vi "LookupFilepath.vi"(0 "Filepath Map":cluster{"Key":string, "Filepath":path}[](array[cluster]), 5 "FileID":string, 11 "error in":errorcluster) -> (15 "error out":errorcluster)   [LabVIEW 2014, in "LinksApplication.lvclass"]
uses:
  LinksApplication.lvclass
panel:
  # "Inputs"
  # "Debug"
  # "Outputs"
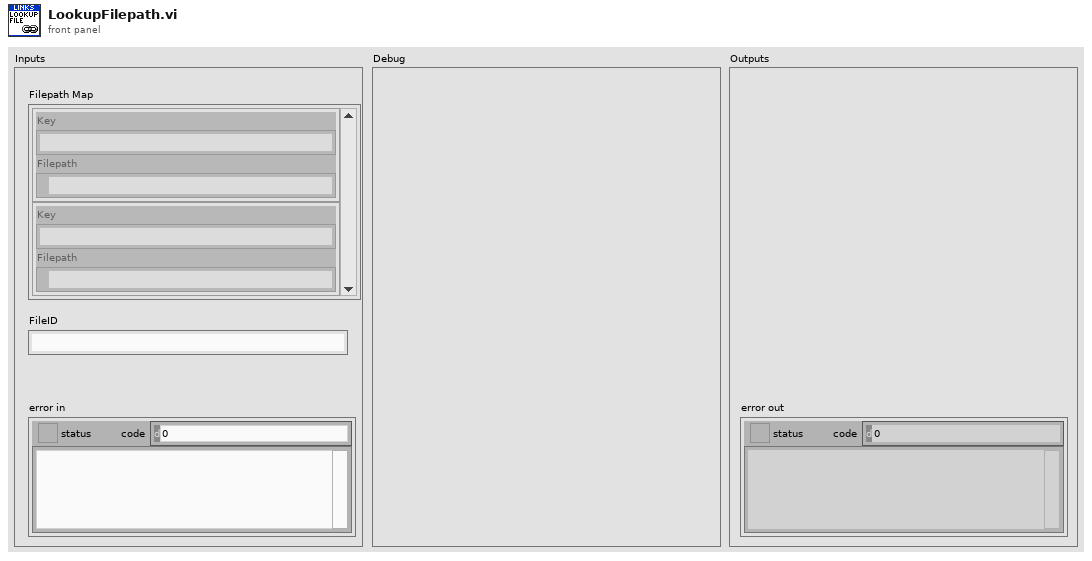
[diagram p1: front panel]
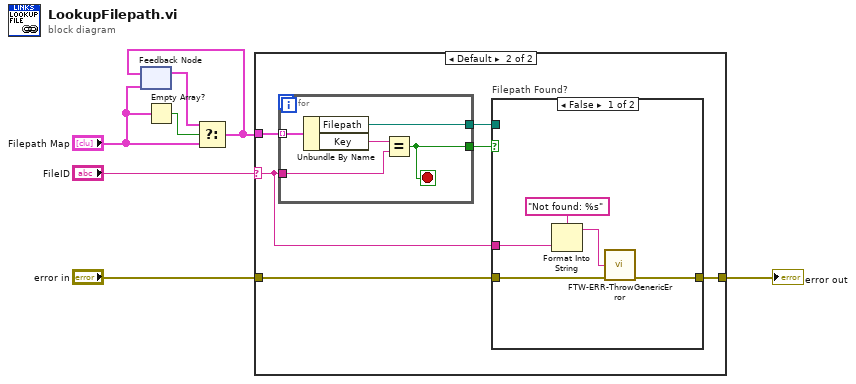
[diagram p0: block diagram]
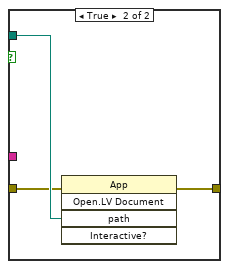
[diagram p3: hidden frame]
diagram:
  n1 = feedback #1("Filepath Map") -> (w4:cluster{"Key":string, "Filepath":path}[])
  n2 = Empty Array?(array="Filepath Map") -> (empty?=w5:bool)
  n3 = Select(t=w4, s=w5, f="Filepath Map") -> (s? t:f=w1:cluster{"Key":string, "Filepath":path}[])
  n4 = feedback-in #1(w1) -> ()
  n5 = case shown="Default" "FileID" {
    selector: "FileID" -> [_ w9]
    tunnel: [w8 w13] -> w7
    tunnel: "error in" -> [w8 w11]
    tunnel: w1 -> [_ w10]
    frame "" {
    }
    frame Default {
      n6 = for {
        tunnel: w10 -> [w27] mode=indexing
        tunnel: w9 -> [w25]
        tunnel: [w24] -> w14
        tunnel: [w23] -> w12
        stop <- w23 stop-if-true
        n7 = Unbundle By Name(w27) -> ("Filepath"=w24:path, "Key"=w26:string)
        n8 = Equal?(x=w26, y=w25) -> (x = y?=w23:bool)
      }
      n9 = case "Filepath Found?" shown="False" w12 {
        tunnel: w14 -> [_ w22]
        tunnel: w11 -> [w19 w21]
        tunnel: [w18 w20] -> w13
        tunnel: w9 -> [w16 _]
        frame False {
          n10 = Format Into String(format string="Not found: %s" ("Error Message"), w16) -> (resulting string=w15:string)  [unwired: 2 in, 1 out]
          n11 = call "FTW-ERR-ThrowGenericError.vi"("Error Message"=w15, "error in"=w19) -> ("error out"=w18:errorcluster)  [unwired: 13 in]
        }
        frame True {
          n12 = invoke class="App" method="Open.LV Document"(error in=w21, "path"=w22) -> (error out=w20:errorcluster)  [unwired: 3 in, 4 out]
        }
      }
    }
  }
  "error out" <- w7
